vi "shm_open.vi"(8 "error in (no error)":errorcluster, 9 "file creation flags":T1[](array[typedef]) items=["O_RDONLY"=0, "O_WRONLY"=1, "O_RDWR"=2, "O_CREAT"=64, "O_EXCL"=128, "O_TRUNC"=512], 10 "permissions (0664)":T2={"owner"={"read"=TRUE, "write"=TRUE, "execute"=FALSE}, "group"={"read"=TRUE, "write"=TRUE, "execute"=FALSE}, "everyone"={"read"=TRUE, "write"=FALSE, "execute"=FALSE}}, 11 "shared memory name":string) -> (0 "error out":errorcluster, 3 "file descriptor":i32)   [LabVIEW 2013, in "Linux RT IPC.C.lvlib"]
doc: "Wrapper VI for Linux function shm_open()."
uses:
  Linux RT IPC.C.lvlib
  Controls/file creation flags.ctl
  Controls/functions.ctl
  SubVIs/path globals.vi
  <vilib>/NI/NI Linux RT Errno/Linux Errno.lvlib
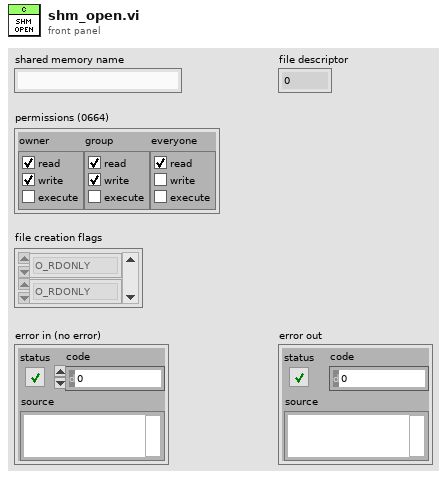
[diagram p1: front panel]
types:
  T1 = typedef "Linux RT IPC.C.lvlib/file creation flags.ctl" = u32
  T2 = cluster{"owner":cluster{"read":bool, "write":bool, "execute":bool}, "group":cluster{"read":bool, "write":bool, "execute":bool}, "everyone":cluster{"read":bool, "write":bool, "execute":bool}}
  T3 = typedef "Linux RT IPC.C.lvlib/functions.ctl" = enum16{"unspecified", "close", "epoll_create", "epoll_ctl", "epoll_wait", "fstat", "ftruncate", "mkfifo", "mmap", "munmap", "open", "read", "shm_open", "shm_unlink", "timerfd_create", "timerfd_settime", "timerfd_gettime", "write", "unlink"}
  T4 = typedef "Linux Errno.lvlib/errno.ctl" = enum16{"NO ERROR", "EPERM", "ENOENT", "ESRCH", "EINTR", "EIO", "ENXIO", "E2BIG", "ENOEXEC", "EBADF", "ECHILD", "EAGAIN", "ENOMEM", "EACCES", "EFAULT", "ENOTBLK", "EBUSY", "EEXIST", "EXDEV", "ENODEV", "ENOTDIR", "EISDIR", "EINVAL", "ENFILE", "EMFILE", "ENOTTY", "ETXTBSY", "EFBIG", "ENOSPC", "ESPIPE", "EROFS", "EMLINK", "EPIPE", "EDOM", "ERANGE", "EDADLK", "ENAMETOOLONG", "ENOLCK", "ENOSYS", "ENOTEMPTY", "ELOOP", "EWOULDBLOCK", "ENOMSG", "EIDRM", "ECHRNG", "EL2NSYNC", "EL3HLT", "EL3RST", "ELNRNG", "EUNATCH", "ENOCSI", "EL2HLT", "EBADE", "EBADR", "EXFULL", "ENOANO", "EBADRQC", "EBADSLT", "EDEADLOCK", "EBFONT", "ENOSTR", "ENODATA", "ETIME", "ENOSR", "ENONET", "ENOPKG", "EREMOTE", "ENOLINK", "EADV", "ESRMNT", "ECOMM", "EPROTO", "EMULTIHOP", "EDOTDOT", "EBADMSG", "EOVERFLOW", "ENOTUNIQ", "EBADFD", "EREMCHG", "ELIBACC", "ELIBBAD", "ELIBSCN", "ELIBMAX", "ELIBEXEC", "ELISEQ", "ERESTART", "ESTRPIPE", "EUSERS", "ENOTSOCK", "EDESTADDRREQ", "EMSGSIZE", "EPROTOTYPE", "ENOPROTOOPT", "EPROTONOSUPPORT", "ESOCKTNOSUPPORT", "EOPNOTSUPP", "EPFNOSUPPORT", "EAFNOSUPPORT", "EADDRINUSE", "EADDRNOTAVAIL", "ENETDOWN", "ENETUNREACH", "ENETRESET", "ECONNABORTED", "ECONNRESET", "ENOBUFS", "EISCONN", "ENOTCONN", "ESHUTDOWN", "ETOOMANYREFS", "ETIMEDOUT", "ECONNREFUSED", "EHOSTDOWN", "EHOSTUNREACH", "EALREADY", "EINPROGRESS", "ESTALE", "EUCLEAN", "ENOTNAM", "ENAVAIL", "EISNAM", "EREMOTEIO", "EDQUOT", "ENOMEDIUM", "EMEDIUMTYPE", "ECANCELED", "ENOKEY", "EKEYEXPIRED", "EKEYREVOKED", "EKEYREJECTED", "EOWNERDEAD", "ENOTRECOVERABLE", "ERFKILL", "EHWPOISON", "UNDEFINED"}
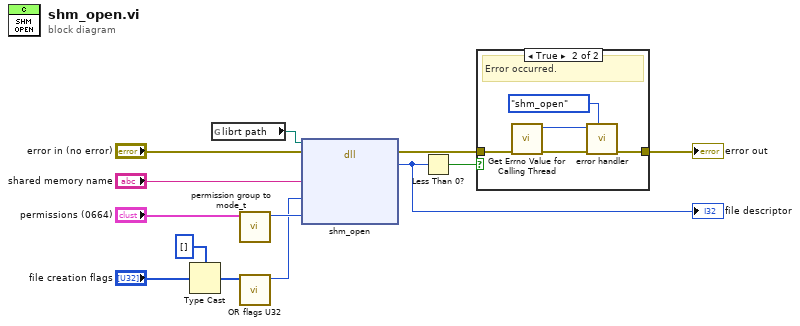
[diagram p0: block diagram]
diagram:
  n1 = Type Cast(type=u32[] [], x="file creation flags") -> (*(type *) &x=w2:u32[])
  n2 = global read "path globals.vi" "librt path"() -> (w6:path)
  n3 = call "permission group to mode_t.vi"("permissions group"="permissions (0664)") -> ("mode_t"=w7:u32)  [unwired: 10 in]
  n4 = call "OR flags U32.vi"("flags"=w2) -> ("OR'ed flags"=w1:u32)  [unwired: 10 in]
  n5 = dll-call lib="?" fn="shm_open"(path in=w6, error in="error in (no error)", "name"="shared memory name", "flags"=w1, "mode"=w7) -> (error out=w9:errorcluster, "fd"=w11:i32)  [unwired: 4 in, 1 out]
  "file descriptor" <- w11
  n6 = Less Than 0?(x=w11) -> (x < 0?=w8:bool)
  n7 = case shown="True" w8 {
    tunnel: w9 -> [w14 w19]
    tunnel: [w14 w17] -> w12
    frame False {
      # "No error."
    }
    frame True {
      # "Error occurred."
      n8 = call <vilib>:"Get Errno Value for Calling Thread.vi"("error in (no error)"=w19) -> ("error out"=w18:errorcluster, "errno"=w16:T4)  [unwired: 9 in]
      n9 = call "error handler.vi"("function (unspecified)"=functions."shm_open", "error in (no error)"=w18, "errno"=w16) -> ("error out"=w17:errorcluster)  [unwired: 8 in]
    }
  }
  "error out" <- w12
